vi "test-PID-test-01-SetSetpoint.vi"() -> (3 "All Passed":bool)   [LabVIEW 2019]
uses:
  <vilib>/Rock Robotics/WPI/ThirdParty/JAS_Junk/TrajLib/Trajectory_Library.lvlib
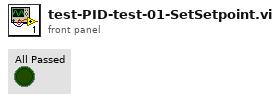
[diagram p1: front panel]
types:
  T1 = typedef "Trajectory_Library.lvlib/PID_CONTROLLER.ctl" = cluster{"Kp":dbl, "Ki":dbl, "Kd":dbl, "Period":dbl, "Max_Integral":dbl, "Min_Integral":dbl, "Max_Input":dbl, "Min_Input":dbl, "Continuous":bool, "PositionError":dbl, "VelocityError":dbl, "PrevError":dbl, "TotalError":dbl, "PositionTolerance":dbl, "VelocityTolerance":dbl, "SetPoint":dbl, "Kf":dbl, "Prev_Deriv":dbl, "Prev_Deriv 2":dbl, "DerivativeFilter":bool, "Min_Output":dbl, "Max_Output":dbl, "Prev_F_P":dbl, "Prev_F_P_2":dbl, "AntiWindupActive":bool, "Measurement":dbl}
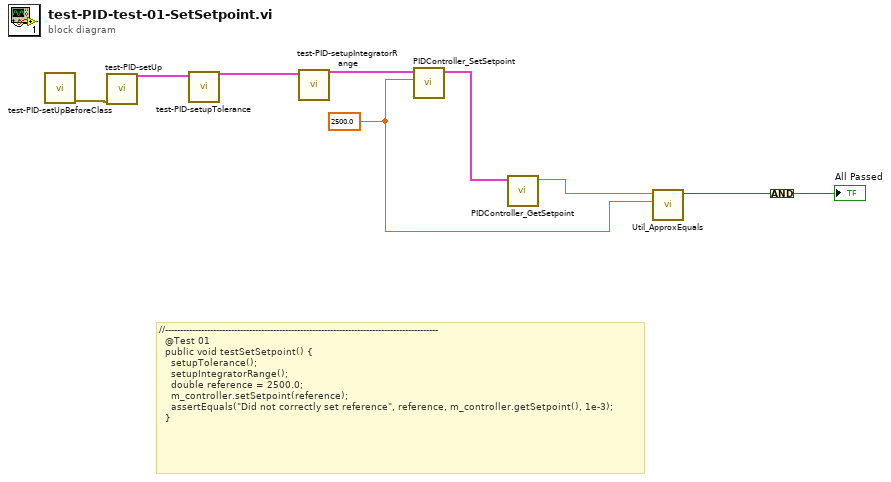
[diagram p0: block diagram]
diagram:
  w4 = 2500.0 ("Setpoint")
  # "//-------------------------------------------------------------------------------------------\n  @Test 01\n  public void testSetSetpoint() {\n    setupTolerance();\n    setupIntegratorRange();\n    double reference = 2500.0;\n    m_controller.setSetpoint(reference);\n    assertEquals(\"Did not correctly set reference\", reference, m_controller.getSetpoint(), 1e-3);\n  }"
  n1 = call "test-PID-setUpBeforeClass.vi"() -> ("error out"=w9:errorcluster)  [unwired: 11 in]
  n2 = call "test-PID-setUp.vi"("error in (no error)"=w9) -> ("PID_CONTROLLER"=w8:T1)  [unwired: 9 in, 1 out]
  n3 = call "test-PID-setupTolerance.vi"("in PID_CONTROLLER"=w8) -> ("out PID_CONTROLLER"=w7:T1)  [unwired: 10 in]
  n4 = call "test-PID-setupIntegratorRange.vi"("in PID_CONTROLLER"=w7) -> ("out PID_CONTROLLER"=w6:T1)  [unwired: 10 in]
  n5 = call <vilib>:"PIDController_SetSetpoint.vi"("Setpoint"=w4, "in PID_CONTROLLER"=w6) -> ("out PID_CONTROLLER"=w2:T1)  [unwired: 9 in]
  n6 = call <vilib>:"PIDController_GetSetpoint.vi"("in PID_CONTROLLER"=w2) -> ("Setpoint"=w5:dbl)  [unwired: 10 in]
  n7 = call <vilib>:"Util_ApproxEquals.vi"("Value 2"=w4, "Value 1"=w5) -> ("ApproxEquals"=w3:bool)  [unwired: 9 in]
  n8 = Compound Arithmetic op=AND(w3) -> (→"All Passed":bool)
